vi "Test Recursive File List.vi"(8 "error in (no error)":errorcluster) -> (0 "error out":errorcluster, 3 "Pass?":bool)   [LabVIEW 2020]
uses:
  G-Unicode/Types/UTF-8 Path/UTF-8 Path.lvclass/UTF-8 Path.ctl
  G-Unicode/Types/UTF-8 String/UTF-8 String.lvclass/UTF-8 String.ctl
  9a10596f-35a4-4ea9-8ab1-c87a4e066f2c.vi
  9a10596f-35a4-4ea9-8ab1-c87a4e066f2c.vi/e59fd3ad-a218-449e-bbf4-8568d0899d6e.vi
  9a10596f-35a4-4ea9-8ab1-c87a4e066f2c.vi/6e4bb66e-265d-408c-9dfe-e7c3a7878e52.vi
  9a10596f-35a4-4ea9-8ab1-c87a4e066f2c.vi/08f180d4-fb41-400e-a869-abb2918b55f1.vi
  9a10596f-35a4-4ea9-8ab1-c87a4e066f2c.vi/5ea8612d-ac84-4b15-a8e8-3f95405e799f.vi
  9a10596f-35a4-4ea9-8ab1-c87a4e066f2c.vi/f443e8ba-b003-43b4-b0bc-fd2b779e8587.vi
  9a10596f-35a4-4ea9-8ab1-c87a4e066f2c.vi/3afc9dd8-07d7-4035-8615-071e8f5e5c27.vi
  9a10596f-35a4-4ea9-8ab1-c87a4e066f2c.vi/c88429ca-af36-48cc-be70-990e2bd8b71c.vi
  9a10596f-35a4-4ea9-8ab1-c87a4e066f2c.vi/73aac6a6-4dac-4660-97c1-8eb854e998dd.vi
  9a10596f-35a4-4ea9-8ab1-c87a4e066f2c.vi/6eb3c72c-ccaf-45c3-aa0c-9c92d51b379f.vi
  9a10596f-35a4-4ea9-8ab1-c87a4e066f2c.vi/d8f6ae1f-7202-4db9-b87a-1f416505b7ed.vi
  G-Unicode/Private/Conversion/Path as UTF-8 Path.vi
  G-Unicode/Private/Conversion/Polymorphic VIs/Path as UTF-8 Path (LabVIEW Path).vi
  G-Unicode/Types/UTF-8 Path/Write Encoded UTF-8 Path.vi
  G-Unicode/Private/Conversion/Path as Encoded Path.vi
  G-Unicode/Private/Conversion/Polymorphic VIs/Path as Encoded Path (UTF-8 Path).vi
  G-Unicode/Types/UTF-8 String/Write Encoded UTF-8 String.vi
  G-Unicode/Private/Library/gu_to_lower_case.vi
  G-Unicode/Private/Conversion/String as Encoded String.vi
  G-Unicode/Private/Conversion/Polymorphic VIs/String as Encoded String (UTF-8 String).vi
  G-Unicode/Private/Conversion/Polymorphic VIs/Path as UTF-8 Path (UTF-8 Path).vi
  9a10596f-35a4-4ea9-8ab1-c87a4e066f2c.vi/08f180d4-fb41-400e-a869-abb2918b55f1.vi/5269e09c-4216-478e-8686-9fb7d38e224a.vi
  9a10596f-35a4-4ea9-8ab1-c87a4e066f2c.vi/08f180d4-fb41-400e-a869-abb2918b55f1.vi/d1f4a45d-6f02-44dd-a40b-2b28d80e6519.vi
  G-Unicode/Private/Library/gu_list_folder.vi
  9a10596f-35a4-4ea9-8ab1-c87a4e066f2c.vi/08f180d4-fb41-400e-a869-abb2918b55f1.vi/d2d8a17d-5f66-4e25-bebc-c290fb73390a.vi
  9a10596f-35a4-4ea9-8ab1-c87a4e066f2c.vi/08f180d4-fb41-400e-a869-abb2918b55f1.vi/f7e6584c-01ed-423f-9bcd-660954191d0d.vi
  9a10596f-35a4-4ea9-8ab1-c87a4e066f2c.vi/5ea8612d-ac84-4b15-a8e8-3f95405e799f.vi/5269e09c-4216-478e-8686-9fb7d38e224a.vi
  9a10596f-35a4-4ea9-8ab1-c87a4e066f2c.vi/5ea8612d-ac84-4b15-a8e8-3f95405e799f.vi/d1f4a45d-6f02-44dd-a40b-2b28d80e6519.vi
  9a10596f-35a4-4ea9-8ab1-c87a4e066f2c.vi/5ea8612d-ac84-4b15-a8e8-3f95405e799f.vi/d2d8a17d-5f66-4e25-bebc-c290fb73390a.vi
  9a10596f-35a4-4ea9-8ab1-c87a4e066f2c.vi/5ea8612d-ac84-4b15-a8e8-3f95405e799f.vi/f7e6584c-01ed-423f-9bcd-660954191d0d.vi
  9a10596f-35a4-4ea9-8ab1-c87a4e066f2c.vi/f443e8ba-b003-43b4-b0bc-fd2b779e8587.vi/bdbb2850-443b-457b-baea-a8ca465ac309.vi
  9a10596f-35a4-4ea9-8ab1-c87a4e066f2c.vi/f443e8ba-b003-43b4-b0bc-fd2b779e8587.vi/12c50203-b387-4b7f-a219-1cc37bee024e.vi
  9a10596f-35a4-4ea9-8ab1-c87a4e066f2c.vi/f443e8ba-b003-43b4-b0bc-fd2b779e8587.vi/79db7a21-11bb-4b22-98c5-d1966ec86c45.vi
  G-Unicode/Types/UTF-8 String/Read Encoded UTF-8 String.vi
  9a10596f-35a4-4ea9-8ab1-c87a4e066f2c.vi/f443e8ba-b003-43b4-b0bc-fd2b779e8587.vi/90888b97-91dc-4a8b-9ef5-bc117a67dfd4.vi
  9a10596f-35a4-4ea9-8ab1-c87a4e066f2c.vi/f443e8ba-b003-43b4-b0bc-fd2b779e8587.vi/1e320fb2-7d21-4fd0-8d77-02d925575486.vi
  9a10596f-35a4-4ea9-8ab1-c87a4e066f2c.vi/f443e8ba-b003-43b4-b0bc-fd2b779e8587.vi/3a50a1cc-fee8-47d0-b63a-e1c29b38961d.vi
  G-Unicode/Private/Conversion/Text as Encoded Path.vi
  G-Unicode/Private/Conversion/Polymorphic VIs/Text as Encoded Path (UTF-8 String).vi
  9a10596f-35a4-4ea9-8ab1-c87a4e066f2c.vi/c88429ca-af36-48cc-be70-990e2bd8b71c.vi/4d3f9d4a-5006-44fd-9ac3-fe6a2ce0b86b.vi
  9a10596f-35a4-4ea9-8ab1-c87a4e066f2c.vi/c88429ca-af36-48cc-be70-990e2bd8b71c.vi/29e5914f-c0b0-4539-b998-9919647c2bfd.vi
  9a10596f-35a4-4ea9-8ab1-c87a4e066f2c.vi/73aac6a6-4dac-4660-97c1-8eb854e998dd.vi/4d3f9d4a-5006-44fd-9ac3-fe6a2ce0b86b.vi
  9a10596f-35a4-4ea9-8ab1-c87a4e066f2c.vi/73aac6a6-4dac-4660-97c1-8eb854e998dd.vi/29e5914f-c0b0-4539-b998-9919647c2bfd.vi
  G-Unicode/Types/UTF-8 Path/New UTF-8 Path.vi
  9a10596f-35a4-4ea9-8ab1-c87a4e066f2c.vi/08f180d4-fb41-400e-a869-abb2918b55f1.vi/5269e09c-4216-478e-8686-9fb7d38e224a.vi/7d24581e-fc49-4179-a43d-a6855ac26a93.vi
  9a10596f-35a4-4ea9-8ab1-c87a4e066f2c.vi/08f180d4-fb41-400e-a869-abb2918b55f1.vi/5269e09c-4216-478e-8686-9fb7d38e224a.vi/036f0c18-93c2-49a9-b76c-9112c06b4f18.vi
  9a10596f-35a4-4ea9-8ab1-c87a4e066f2c.vi/08f180d4-fb41-400e-a869-abb2918b55f1.vi/5269e09c-4216-478e-8686-9fb7d38e224a.vi/a2fd6c11-d594-45c9-8624-1f0a1df69df3.vi
  9a10596f-35a4-4ea9-8ab1-c87a4e066f2c.vi/08f180d4-fb41-400e-a869-abb2918b55f1.vi/5269e09c-4216-478e-8686-9fb7d38e224a.vi/1fd3173e-d32e-42cb-8f0d-819132eb8e27.vi
  G-Unicode/Private/Conversion/Text as Encoded String.vi
  G-Unicode/Private/Conversion/Polymorphic VIs/Text as Encoded String (UTF-8 Path).vi
  9a10596f-35a4-4ea9-8ab1-c87a4e066f2c.vi/08f180d4-fb41-400e-a869-abb2918b55f1.vi/d2d8a17d-5f66-4e25-bebc-c290fb73390a.vi/3a31b270-3bb6-4c58-a256-c5fcc2c98f09.vi
  9a10596f-35a4-4ea9-8ab1-c87a4e066f2c.vi/08f180d4-fb41-400e-a869-abb2918b55f1.vi/d2d8a17d-5f66-4e25-bebc-c290fb73390a.vi/0ec5df2d-ef9b-4f84-a6a8-ffcedd45c4dc.vi
  9a10596f-35a4-4ea9-8ab1-c87a4e066f2c.vi/5ea8612d-ac84-4b15-a8e8-3f95405e799f.vi/5269e09c-4216-478e-8686-9fb7d38e224a.vi/7d24581e-fc49-4179-a43d-a6855ac26a93.vi
  9a10596f-35a4-4ea9-8ab1-c87a4e066f2c.vi/5ea8612d-ac84-4b15-a8e8-3f95405e799f.vi/5269e09c-4216-478e-8686-9fb7d38e224a.vi/036f0c18-93c2-49a9-b76c-9112c06b4f18.vi
  9a10596f-35a4-4ea9-8ab1-c87a4e066f2c.vi/5ea8612d-ac84-4b15-a8e8-3f95405e799f.vi/5269e09c-4216-478e-8686-9fb7d38e224a.vi/a2fd6c11-d594-45c9-8624-1f0a1df69df3.vi
  9a10596f-35a4-4ea9-8ab1-c87a4e066f2c.vi/5ea8612d-ac84-4b15-a8e8-3f95405e799f.vi/5269e09c-4216-478e-8686-9fb7d38e224a.vi/1fd3173e-d32e-42cb-8f0d-819132eb8e27.vi
  9a10596f-35a4-4ea9-8ab1-c87a4e066f2c.vi/5ea8612d-ac84-4b15-a8e8-3f95405e799f.vi/d2d8a17d-5f66-4e25-bebc-c290fb73390a.vi/3a31b270-3bb6-4c58-a256-c5fcc2c98f09.vi
  9a10596f-35a4-4ea9-8ab1-c87a4e066f2c.vi/5ea8612d-ac84-4b15-a8e8-3f95405e799f.vi/d2d8a17d-5f66-4e25-bebc-c290fb73390a.vi/0ec5df2d-ef9b-4f84-a6a8-ffcedd45c4dc.vi
  G-Unicode/Private/Library/gu_string_subset.vi
  9a10596f-35a4-4ea9-8ab1-c87a4e066f2c.vi/f443e8ba-b003-43b4-b0bc-fd2b779e8587.vi/90888b97-91dc-4a8b-9ef5-bc117a67dfd4.vi/5269e09c-4216-478e-8686-9fb7d38e224a.vi
  9a10596f-35a4-4ea9-8ab1-c87a4e066f2c.vi/f443e8ba-b003-43b4-b0bc-fd2b779e8587.vi/90888b97-91dc-4a8b-9ef5-bc117a67dfd4.vi/d1f4a45d-6f02-44dd-a40b-2b28d80e6519.vi
  9a10596f-35a4-4ea9-8ab1-c87a4e066f2c.vi/f443e8ba-b003-43b4-b0bc-fd2b779e8587.vi/90888b97-91dc-4a8b-9ef5-bc117a67dfd4.vi/d2d8a17d-5f66-4e25-bebc-c290fb73390a.vi
  9a10596f-35a4-4ea9-8ab1-c87a4e066f2c.vi/f443e8ba-b003-43b4-b0bc-fd2b779e8587.vi/90888b97-91dc-4a8b-9ef5-bc117a67dfd4.vi/f7e6584c-01ed-423f-9bcd-660954191d0d.vi
  9a10596f-35a4-4ea9-8ab1-c87a4e066f2c.vi/f443e8ba-b003-43b4-b0bc-fd2b779e8587.vi/1e320fb2-7d21-4fd0-8d77-02d925575486.vi/5269e09c-4216-478e-8686-9fb7d38e224a.vi
  9a10596f-35a4-4ea9-8ab1-c87a4e066f2c.vi/f443e8ba-b003-43b4-b0bc-fd2b779e8587.vi/1e320fb2-7d21-4fd0-8d77-02d925575486.vi/d1f4a45d-6f02-44dd-a40b-2b28d80e6519.vi
  9a10596f-35a4-4ea9-8ab1-c87a4e066f2c.vi/f443e8ba-b003-43b4-b0bc-fd2b779e8587.vi/1e320fb2-7d21-4fd0-8d77-02d925575486.vi/d2d8a17d-5f66-4e25-bebc-c290fb73390a.vi
  9a10596f-35a4-4ea9-8ab1-c87a4e066f2c.vi/f443e8ba-b003-43b4-b0bc-fd2b779e8587.vi/1e320fb2-7d21-4fd0-8d77-02d925575486.vi/f7e6584c-01ed-423f-9bcd-660954191d0d.vi
  G-Unicode/Private/Conversion/Polymorphic VIs/String as Encoded String (LabVIEW String).vi
  9a10596f-35a4-4ea9-8ab1-c87a4e066f2c.vi/f443e8ba-b003-43b4-b0bc-fd2b779e8587.vi/3a50a1cc-fee8-47d0-b63a-e1c29b38961d.vi/5269e09c-4216-478e-8686-9fb7d38e224a.vi
  9a10596f-35a4-4ea9-8ab1-c87a4e066f2c.vi/f443e8ba-b003-43b4-b0bc-fd2b779e8587.vi/3a50a1cc-fee8-47d0-b63a-e1c29b38961d.vi/d1f4a45d-6f02-44dd-a40b-2b28d80e6519.vi
  9a10596f-35a4-4ea9-8ab1-c87a4e066f2c.vi/f443e8ba-b003-43b4-b0bc-fd2b779e8587.vi/3a50a1cc-fee8-47d0-b63a-e1c29b38961d.vi/d2d8a17d-5f66-4e25-bebc-c290fb73390a.vi
  9a10596f-35a4-4ea9-8ab1-c87a4e066f2c.vi/f443e8ba-b003-43b4-b0bc-fd2b779e8587.vi/3a50a1cc-fee8-47d0-b63a-e1c29b38961d.vi/f7e6584c-01ed-423f-9bcd-660954191d0d.vi
  G-Unicode/Private/Conversion/Polymorphic VIs/Text as Encoded String (UTF-8 String).vi
  G-Unicode/Private/Conversion/Polymorphic VIs/Text as Encoded String (LabVIEW String).vi
  G-Unicode/Private/Library/gu_search_split_string.vi
  G-Unicode/Private/Memory/Copy String.vi
  9a10596f-35a4-4ea9-8ab1-c87a4e066f2c.vi/f443e8ba-b003-43b4-b0bc-fd2b779e8587.vi/90888b97-91dc-4a8b-9ef5-bc117a67dfd4.vi/5269e09c-4216-478e-8686-9fb7d38e224a.vi/7d24581e-fc49-4179-a43d-a6855ac26a93.vi
  9a10596f-35a4-4ea9-8ab1-c87a4e066f2c.vi/f443e8ba-b003-43b4-b0bc-fd2b779e8587.vi/90888b97-91dc-4a8b-9ef5-bc117a67dfd4.vi/5269e09c-4216-478e-8686-9fb7d38e224a.vi/036f0c18-93c2-49a9-b76c-9112c06b4f18.vi
  9a10596f-35a4-4ea9-8ab1-c87a4e066f2c.vi/f443e8ba-b003-43b4-b0bc-fd2b779e8587.vi/90888b97-91dc-4a8b-9ef5-bc117a67dfd4.vi/5269e09c-4216-478e-8686-9fb7d38e224a.vi/a2fd6c11-d594-45c9-8624-1f0a1df69df3.vi
  9a10596f-35a4-4ea9-8ab1-c87a4e066f2c.vi/f443e8ba-b003-43b4-b0bc-fd2b779e8587.vi/90888b97-91dc-4a8b-9ef5-bc117a67dfd4.vi/5269e09c-4216-478e-8686-9fb7d38e224a.vi/1fd3173e-d32e-42cb-8f0d-819132eb8e27.vi
  9a10596f-35a4-4ea9-8ab1-c87a4e066f2c.vi/f443e8ba-b003-43b4-b0bc-fd2b779e8587.vi/90888b97-91dc-4a8b-9ef5-bc117a67dfd4.vi/d2d8a17d-5f66-4e25-bebc-c290fb73390a.vi/3a31b270-3bb6-4c58-a256-c5fcc2c98f09.vi
  9a10596f-35a4-4ea9-8ab1-c87a4e066f2c.vi/f443e8ba-b003-43b4-b0bc-fd2b779e8587.vi/90888b97-91dc-4a8b-9ef5-bc117a67dfd4.vi/d2d8a17d-5f66-4e25-bebc-c290fb73390a.vi/0ec5df2d-ef9b-4f84-a6a8-ffcedd45c4dc.vi
  9a10596f-35a4-4ea9-8ab1-c87a4e066f2c.vi/f443e8ba-b003-43b4-b0bc-fd2b779e8587.vi/1e320fb2-7d21-4fd0-8d77-02d925575486.vi/5269e09c-4216-478e-8686-9fb7d38e224a.vi/7d24581e-fc49-4179-a43d-a6855ac26a93.vi
  9a10596f-35a4-4ea9-8ab1-c87a4e066f2c.vi/f443e8ba-b003-43b4-b0bc-fd2b779e8587.vi/1e320fb2-7d21-4fd0-8d77-02d925575486.vi/5269e09c-4216-478e-8686-9fb7d38e224a.vi/036f0c18-93c2-49a9-b76c-9112c06b4f18.vi
  9a10596f-35a4-4ea9-8ab1-c87a4e066f2c.vi/f443e8ba-b003-43b4-b0bc-fd2b779e8587.vi/1e320fb2-7d21-4fd0-8d77-02d925575486.vi/5269e09c-4216-478e-8686-9fb7d38e224a.vi/a2fd6c11-d594-45c9-8624-1f0a1df69df3.vi
  9a10596f-35a4-4ea9-8ab1-c87a4e066f2c.vi/f443e8ba-b003-43b4-b0bc-fd2b779e8587.vi/1e320fb2-7d21-4fd0-8d77-02d925575486.vi/5269e09c-4216-478e-8686-9fb7d38e224a.vi/1fd3173e-d32e-42cb-8f0d-819132eb8e27.vi
  9a10596f-35a4-4ea9-8ab1-c87a4e066f2c.vi/f443e8ba-b003-43b4-b0bc-fd2b779e8587.vi/1e320fb2-7d21-4fd0-8d77-02d925575486.vi/d2d8a17d-5f66-4e25-bebc-c290fb73390a.vi/3a31b270-3bb6-4c58-a256-c5fcc2c98f09.vi
  9a10596f-35a4-4ea9-8ab1-c87a4e066f2c.vi/f443e8ba-b003-43b4-b0bc-fd2b779e8587.vi/1e320fb2-7d21-4fd0-8d77-02d925575486.vi/d2d8a17d-5f66-4e25-bebc-c290fb73390a.vi/0ec5df2d-ef9b-4f84-a6a8-ffcedd45c4dc.vi
  9a10596f-35a4-4ea9-8ab1-c87a4e066f2c.vi/f443e8ba-b003-43b4-b0bc-fd2b779e8587.vi/3a50a1cc-fee8-47d0-b63a-e1c29b38961d.vi/5269e09c-4216-478e-8686-9fb7d38e224a.vi/7d24581e-fc49-4179-a43d-a6855ac26a93.vi
  9a10596f-35a4-4ea9-8ab1-c87a4e066f2c.vi/f443e8ba-b003-43b4-b0bc-fd2b779e8587.vi/3a50a1cc-fee8-47d0-b63a-e1c29b38961d.vi/5269e09c-4216-478e-8686-9fb7d38e224a.vi/036f0c18-93c2-49a9-b76c-9112c06b4f18.vi
  9a10596f-35a4-4ea9-8ab1-c87a4e066f2c.vi/f443e8ba-b003-43b4-b0bc-fd2b779e8587.vi/3a50a1cc-fee8-47d0-b63a-e1c29b38961d.vi/5269e09c-4216-478e-8686-9fb7d38e224a.vi/a2fd6c11-d594-45c9-8624-1f0a1df69df3.vi
  9a10596f-35a4-4ea9-8ab1-c87a4e066f2c.vi/f443e8ba-b003-43b4-b0bc-fd2b779e8587.vi/3a50a1cc-fee8-47d0-b63a-e1c29b38961d.vi/5269e09c-4216-478e-8686-9fb7d38e224a.vi/1fd3173e-d32e-42cb-8f0d-819132eb8e27.vi
  9a10596f-35a4-4ea9-8ab1-c87a4e066f2c.vi/f443e8ba-b003-43b4-b0bc-fd2b779e8587.vi/3a50a1cc-fee8-47d0-b63a-e1c29b38961d.vi/d2d8a17d-5f66-4e25-bebc-c290fb73390a.vi/3a31b270-3bb6-4c58-a256-c5fcc2c98f09.vi
  9a10596f-35a4-4ea9-8ab1-c87a4e066f2c.vi/f443e8ba-b003-43b4-b0bc-fd2b779e8587.vi/3a50a1cc-fee8-47d0-b63a-e1c29b38961d.vi/d2d8a17d-5f66-4e25-bebc-c290fb73390a.vi/0ec5df2d-ef9b-4f84-a6a8-ffcedd45c4dc.vi
  G-Unicode/Private/Memory/Copy String.vi/4d47babd-4a2d-4eb7-b91b-7e707d692665.vi
  G-Unicode/Private/Library/gu_free.vi
  G-Unicode/File IO/Path to Short Name.vi
  G-Unicode/Private/Memory/Copy String Array.vi
  G-Unicode/Private/Library/gu_strlen.vi
  G-Unicode/Types/UTF-8 String/UTF-8 String.lvclass
  G-Unicode/Types/UTF-8 Path/UTF-8 Path.lvclass
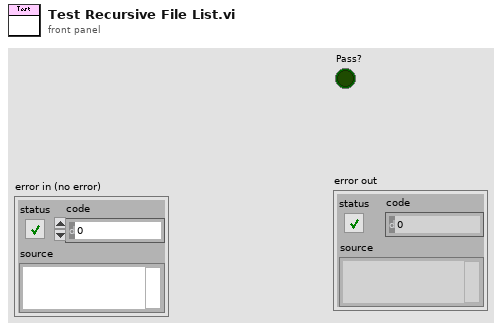
[diagram p1: front panel]
types:
  T1 = typedef "G-Unicode.lvlib/Encoded UTF-8 Path.ctl" = path
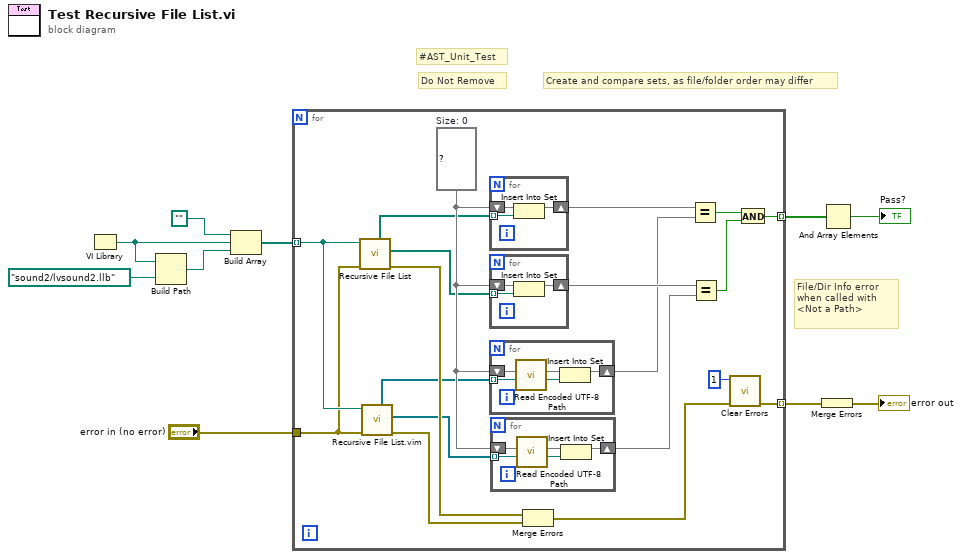
[diagram p0: block diagram]
diagram:
  # "Create and compare sets, as file/folder order may differ"
  # "File/Dir Info error when called with <Not a Path>"
  # "Do Not Remove"
  # "#AST_Unit_Test"
  n1 = VI Library() -> (path=w3:path)
  n2 = Build Path(base path=w3, name or relative path=path "sound2/lvsound2.llb") -> (appended path=w2:path)
  n3 = Build Array(path "", w3, w2) -> (w6:path[])
  n4 = for {
    tunnel: w6 -> [w29] mode=indexing
    tunnel: [w22] -> w9 mode=indexing
    tunnel: "error in (no error)" -> [w28]
    tunnel: [w18] -> w8 mode=indexing
    w27 = set{path} {}  # Size: 0
    n5 = call <vilib>:"Recursive File List.vi"("error in (no error)"=w28, "Folder Path"=w29) -> ("error out"=w21:errorcluster, "All Files in Dir"=w13:path[], "All Folders"=w14:path[])  [unwired: 5 in, 2 out]
    n6 = call "Recursive File List.vim"("error in (no error)"=w28, "Folder Path"=w29) -> ("error out"=w20:errorcluster, "All Files in Dir"=w15:refnum<class "UTF-8 Path.lvclass">[], "All Folders"=w16:refnum<class "UTF-8 Path.lvclass">[])  [unwired: 5 in, 2 out]
    n7 = for {
      tunnel: w14 -> [w43] mode=indexing
      shift-right: [w41] -> w11
      shift-left: w27 -> [w42]
      n8 = Insert Into Set(10:w43, 11:w42) -> (3:w41:set{path})  [unwired: 1 out]
    }
    n9 = for {
      tunnel: w13 -> [w40] mode=indexing
      shift-right: [w38] -> w26
      shift-left: w27 -> [w39]
      n10 = Insert Into Set(10:w40, 11:w39) -> (3:w38:set{path})  [unwired: 1 out]
    }
    n11 = for {
      tunnel: w16 -> [w37] mode=indexing
      shift-right: [w35] -> w12
      shift-left: w27 -> [w36]
      n12 = call "Read Encoded UTF-8 Path.vi"("UTF-8 Path"=w37) -> ("Encoded UTF-8 Path"=w34:T1)  [unwired: 10 in]
      n13 = Insert Into Set(10:w34, 11:w36) -> (3:w35:set{path})  [unwired: 1 out]
    }
    n14 = for {
      tunnel: w15 -> [w33] mode=indexing
      shift-right: [w31] -> w25
      shift-left: w27 -> [w32]
      n15 = call "Read Encoded UTF-8 Path.vi"("UTF-8 Path"=w33) -> ("Encoded UTF-8 Path"=w30:T1)  [unwired: 10 in]
      n16 = Insert Into Set(10:w30, 11:w32) -> (3:w31:set{path})  [unwired: 1 out]
    }
    n17 = Merge Errors(w21, w20) -> (w19:errorcluster)
    n18 = Equal?(x=w11, y=w12) -> (x = y?=w24:bool)
    n19 = Equal?(x=w26, y=w25) -> (x = y?=w23:bool)
    n20 = call <vilib>:"Clear Errors.vi"("error in (no error)"=w19, "specific error code to clear (0: all)"=1) -> ("error out"=w18:errorcluster)  [unwired: 4 in, 1 out]
    n21 = And(x=w24, y=w23) -> (x .and. y?=w22:bool)
  }
  n22 = Merge Errors(w8) -> (→"error out":errorcluster)
  n23 = And Array Elements(Boolean array=w9) -> (logical AND=→"Pass?":bool)
